vi "Append Data.vi"(0 "Socket Auto Connect in":refnum<class "Socket Auto Connect.lvclass">, 5 "String to Append":string, 9 "Scroll (T)":bool=TRUE, 11 "Return (T)":bool=TRUE) -> (14 "Socket Auto Connect out":refnum<class "Socket Auto Connect.lvclass">, 19 "Resulting String":string)   [LabVIEW 2016, in "Socket Auto Connect.lvclass"]
uses:
  Socket Auto Connect.lvclass
  Socket Auto Connect.lvclass/Socket Auto Connect.ctl
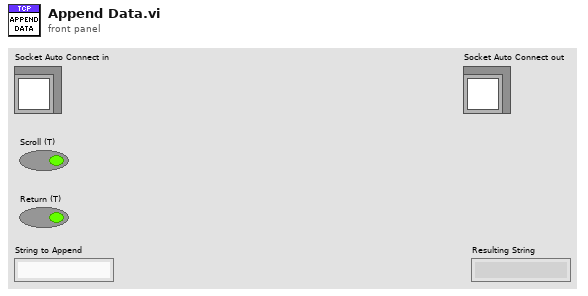
[diagram p1: front panel]
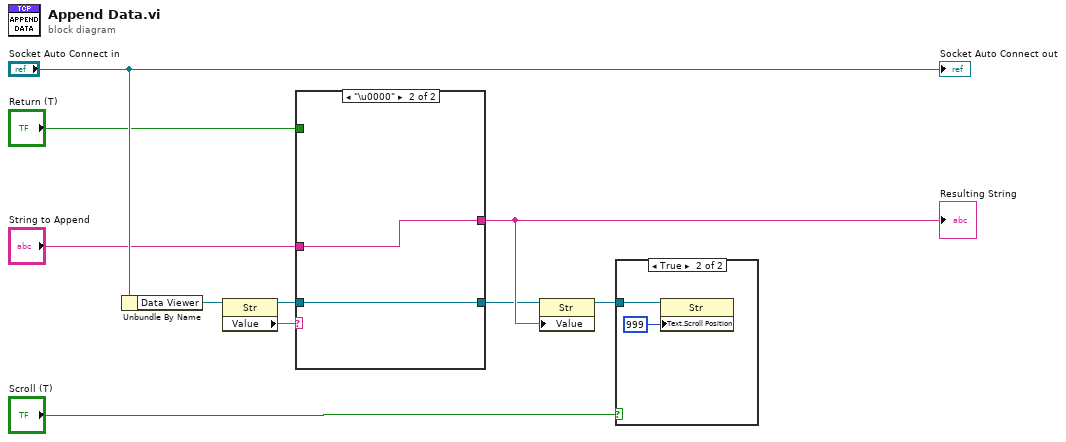
[diagram p0: block diagram]
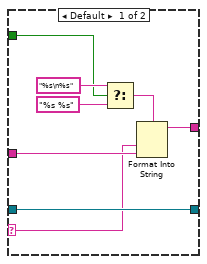
[diagram p2: hidden frame]
diagram:
  n1 = Unbundle By Name("Socket Auto Connect in") -> ("Data Viewer"=w4:refnum<vi>)
  n2 = property class="Str"(reference=w4) -> (reference out=w3:refnum<vi>, "Value"=w1:string)  [unwired: 1 in, 1 out]
  n3 = case shown="\"\"" w1 {
    selector: w1 -> [w11 _]
    tunnel: [w18 w19] -> w9
    tunnel: "String to Append" -> [w17 w19]
    tunnel: "Return (T)" -> [w13 _]
    tunnel: w3 -> [w12 w20]
    tunnel: [w12 w20] -> w2
    frame Default {
      n4 = Select(t="%s\n%s" ("format string"), s=w13, f="%s %s" ("format string")) -> (s? t:f=w15:string)
      n5 = Format Into String(format string=w15, w11, w17) -> (resulting string=w18:string)  [unwired: 2 in, 1 out]
    }
    frame "\u0000" {
    }
  }
  "Resulting String" <- w9
  n6 = property class="Str"(reference=w2, "Value"=w9) -> (reference out=w6:refnum<vi>)  [unwired: 1 in, 1 out]
  n7 = case shown="True" "Scroll (T)" {
    tunnel: w6 -> [_ w22]
    frame False {
    }
    frame True {
      n8 = property class="Str"(reference=w22, "Text.Scroll Position"=u32 999) -> ()  [unwired: 1 in, 2 out]
    }
  }
  "Socket Auto Connect out" <- "Socket Auto Connect in"
